vi "Get Image Size.vi"(8 "error in (no error)":errorcluster, 11 "Buffer in":refnum<class "Buffer.lvclass">) -> (0 "error out":errorcluster, 2 "Image Size":T1, 3 "Buffer":refnum<class "Buffer.lvclass">)   [LabVIEW 2020, in "Buffer.lvclass"]
doc: "Get the dimensions of the image data in the buffer."
uses:
  Buffer.lvclass
  Image Size.ctl
  Buffer.lvclass/Buffer.ctl
  <vilib>/Utility/error.llb/Error Cluster From Error Code.vi
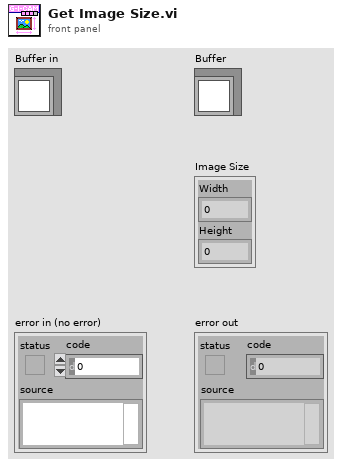
[diagram p1: front panel]
types:
  T1 = typedef "Buffer.lvclass/Image Size.ctl" = cluster{"Width":u16, "Height":u16}
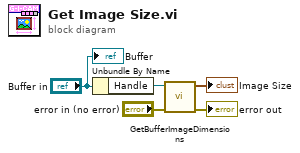
[diagram p0: block diagram]
diagram:
  n1 = Unbundle By Name("Buffer in") -> ("Handle"=w1:refnum<data-value>)
  n2 = call "GetBufferImageDimensions.vi"("error in (no error)"="error in (no error)", "Data Value Reference in"=w1) -> ("error out"=→"error out":errorcluster, "Dims"=→"Image Size":T1)  [unwired: 8 in]
  "Buffer" <- "Buffer in"
